vi "Process Kalibrier Info Cluster.vi"(7 "show Status even if no Error":bool, 8 "Sprachliste":string[][](array[string]), 11 "Kalibrier Info-Cluster in":T1) -> (2 "Fehler":bool, 3 "String":string)   [LabVIEW 2020, in "Linearisierung v2.lvlib" / "SpanEinstellungen.lvlib"]
uses:
  SpanEinstellungen.lvlib
  Kalibrier Info Cluster.ctl
  Sprachverwaltung/Sprachverwaltung.lvlib
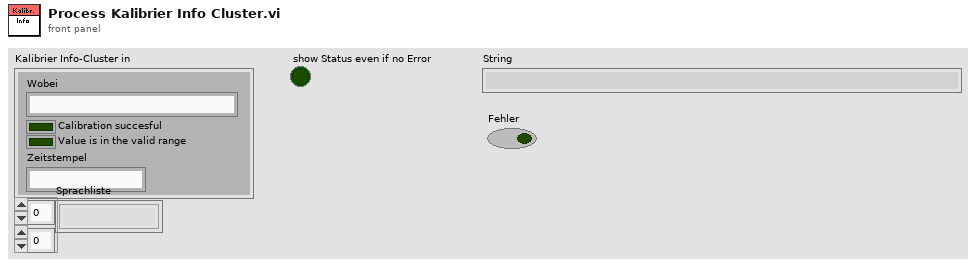
[diagram p1: front panel]
types:
  T1 = typedef "Linearisierung v2.lvlib/SpanEinstellungen.lvlib/Kalibrier Info Cluster.ctl" = cluster{"Wobei":string, "Calibration succesful":bool, "Value is in the valid range":bool, "Zeitstempel":string}
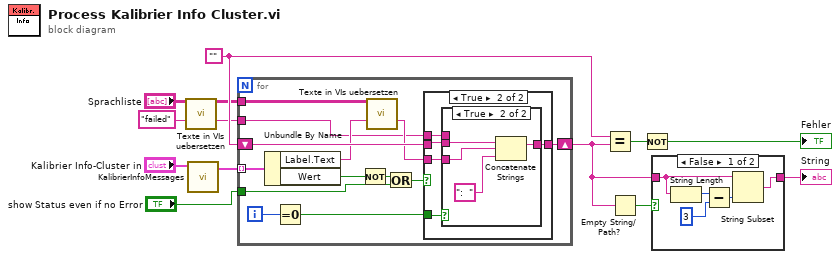
[diagram p0: block diagram]
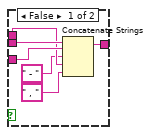
[diagram p4: hidden frame]
diagram:
  w12 = ""
  n1 = call "Texte in VIs uebersetzen.vi"("Sprachliste"="Sprachliste", "String zum Übersetzen"="failed" ("String")) -> ("Sprachliste out"=w7:string[][], "String zum Übersetzen"=w5:string)  [unwired: 9 in, 3 out]
  n2 = call "KalibrierInfoMessages.vi"("Kalibrier Info-Cluster in"="Kalibrier Info-Cluster in") -> ("Kalibrier Info Messages Array"=w9:cluster{"Label.Text":string, "Wert":bool}[])  [unwired: 9 in, 1 out]
  n3 = for {
    tunnel: w9 -> [w26] mode=indexing
    shift-right: [w24] -> w2
    shift-left: w12 -> [w23]
    tunnel: w7 -> [w22]
    tunnel: w5 -> [w19]
    tunnel: "show Status even if no Error" -> [w15]
    i -> [w18]
    n4 = Unbundle By Name(w26) -> ("Label.Text"=w21:string, "Wert"=w25:bool)
    n5 = Equal To 0?(x=w18) -> (x = 0?=w17:bool)
    n6 = Not(x=w25) -> (.not. x?=w14:bool)
    n7 = call "Texte in VIs uebersetzen.vi"("Sprachliste"=w22, "String zum Übersetzen"=w21) -> ("String zum Übersetzen"=w20:string)  [unwired: 9 in, 4 out]
    n8 = Or(x=w14, y=w15) -> (x .or. y?=w16:bool)
    n9 = case shown="True" w16 {
      tunnel: w20 -> [_ w32]
      tunnel: [w27 w31] -> w24
      tunnel: w23 -> [w27 w30]
      tunnel: w19 -> [_ w29]
      tunnel: w17 -> [_ w28]
      frame False {
      }
      frame True {
        n10 = case shown="True" w28 {
          tunnel: w32 -> [w38 w42]
          tunnel: [w37 w41] -> w31
          tunnel: w30 -> [w36 w40]
          tunnel: w29 -> [w35 _]
          frame False {
            n11 = Concatenate Strings(w36, w38, " - " ("String"), w35, " , " ("String")) -> (w37:string)
          }
          frame True {
            n12 = Concatenate Strings(w40, w42, ":  " ("String")) -> (w41:string)
          }
        }
      }
    }
  }
  n13 = Equal?(x=w12, y=w2) -> (x = y?=w11:bool)
  n14 = Empty String/Path?(string/path=w2) -> (empty?=w4:bool)
  n15 = Not(x=w11) -> (.not. x?=→"Fehler":bool)
  n16 = case shown="False" w4 {
    tunnel: [w46 w48] -> w3
    tunnel: w2 -> [w47 w48]
    frame False {
      n17 = String Length(string=w47) -> (length=w45:i32)
      n18 = Subtract(x=w45, y=3 ("x")) -> (x-y=w44:i32)
      n19 = String Subset(string=w47, length (rest)=w44) -> (substring=w46:string)  [unwired: 1 in]
    }
    frame True {
    }
  }
  "String" <- w3
